vi "Output (subVI).vi"(1 "High Period (us)":u32, 2 "Low Period (us)":u32) -> (0 "Output 0":bool)   [LabVIEW 2016]
doc: "This subVI supports a PWM output application. It translates the Low Pulse and High Pulse inputs to the number of microseconds that the output PWM should stay low and high, respectively."
panel:
  # "This subVI supports a PWM output application.  It translates the Low Pulse and High Pulse inputs to the number of microseconds that the output PWM should stay low and high, respectively."
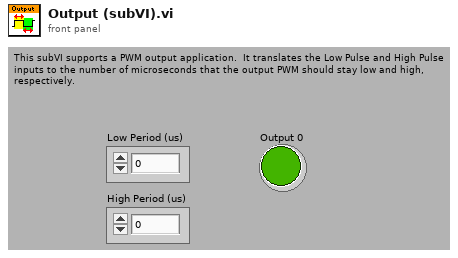
[diagram p1: front panel]
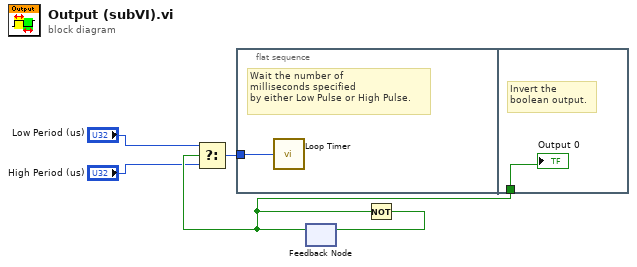
[diagram p0: block diagram]
diagram:
  n1 = flat-sequence {
    tunnel: w5 -> [w6]
    tunnel: w3 -> [w7]
    frame #0 {
      # "Wait the number of \nmilliseconds specified\nby either Low Pulse or High Pulse."
      n2 = call "Loop Timer"("Count(uSec)"=w6) -> ()  [unwired: 1 out]
    }
    frame #1 {
      # "Invert the \nboolean output."
      "Output 0" <- w7
    }
  }
  n3 = feedback #1() -> (w3:bool)  [unwired: 1 out]
  n4 = Select(t="Low Period (us)", s=w3, f="High Period (us)") -> (s? t:f=w5:u32)
  n5 = Not(x=w3) -> (.not. x?=w4:bool)
  n6 = feedback-in #1(w4) -> ()
